vi "XL320_Query Voltage.vi"(8 "error in (no error)":errorcluster, 10 "Motor ID (0)":u8, 11 "VISA resource name":refnum<visa-resource-name>) -> (0 "error out":errorcluster, 2 "Voltage (V)":sgl, 3 "VISA resource name out":refnum<visa-resource-name>)   [LabVIEW 2017, in "Dynamixel XL320.lvlib"]
doc: "Gets the motor's voltage."
uses:
  <instrlib>/Dynamixel XL320 (Drivers instrument)/Dynamixel XL320.lvlib
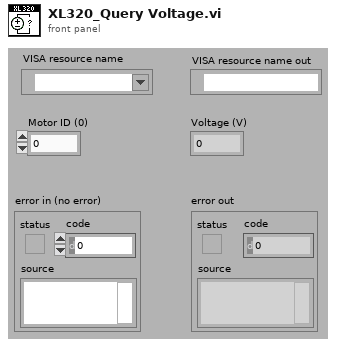
[diagram p1: front panel]
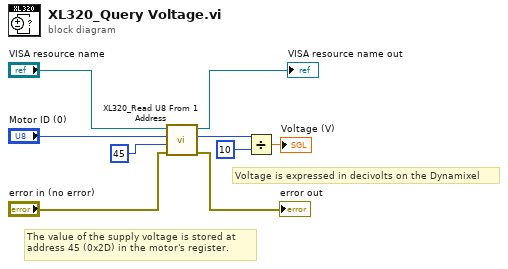
[diagram p0: block diagram]
diagram:
  # "The value of the supply voltage is stored at \naddress 45 (0x2D) in the motor's register."
  # "Voltage is expressed in decivolts on the Dynamixel"
  n1 = call <instrlib>:"XL320_Read U8 From 1 Address.vi"("Error in (no error)"="error in (no error)", "Address number (0)"=u8 45 ("Address # DEC"), "Motor ID (0)"="Motor ID (0)", "VISA resource name"="VISA resource name") -> ("error out"=→"error out":errorcluster, "Data"=w3:u8, "VISA resource name out"=→"VISA resource name out":refnum<visa-resource-name>)  [unwired: 5 in]
  n2 = Divide(x=w3, y=u8 10) -> (x/y=→"Voltage (V)":dbl)
